vi "SRV_Select a String Dialog.vi"(10 "String List":string[](array[string]), 11 "Prompt (Select one item.)":string="Select one item.") -> (0 "Cancelled?":bool, 2 "Selected String":string)   [LabVIEW 2014]
doc: "This dialog allows the user to select exactly one string from an array of input strings.\n\nAuthor: Mike Schultz"
panel:
  in  "Cancel":bool
  in  "OK":bool
  in  "Listbox":i32(listbox)
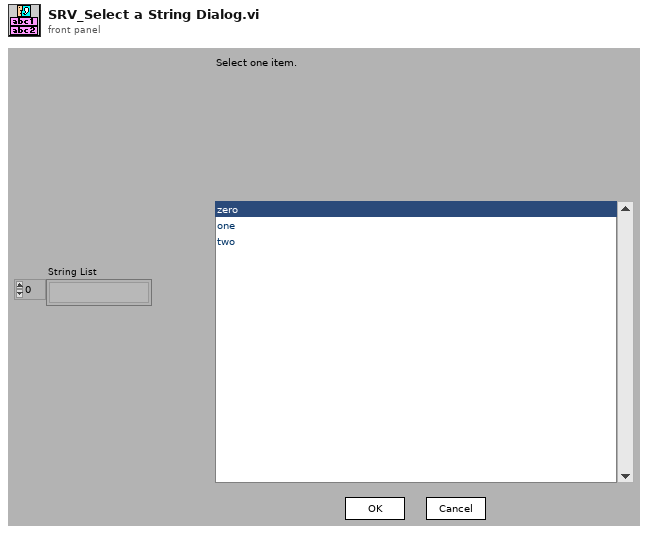
[diagram p1: front panel]
types:
  T1 = cluster{"top":i16, "left":i16, "bottom":i16, "right":i16}
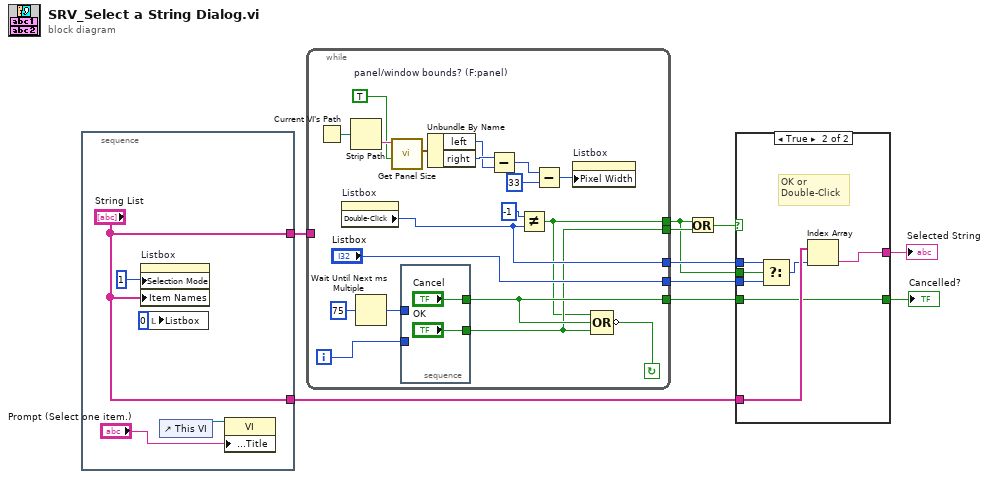
[diagram p0: block diagram]
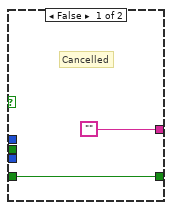
[diagram p2: hidden frame]
diagram:
  n1 = stacked-sequence {
    tunnel: ["String List"] -> w10
    tunnel: ["String List"] -> w1
    frame #0 {
      n2 = property on="Listbox" class="LstBox (strict)"("Selection Mode"=1, "Item Names"="String List") -> ()  [unwired: 2 in, 2 out]
      n3 = local write "Listbox"(0 ("Listbox")) -> ()
      n4 = control-ref of="This VI"() -> (w12:refnum<vi>)
      n5 = property class="VI"(reference=w12, "Front Panel.Title"="Prompt (Select one item.)") -> ()  [unwired: 1 in, 2 out]
    }
  }
  n6 = while {
    tunnel: w1 -> [_]
    tunnel: [w27] -> w3
    tunnel: [w26] -> w2
    tunnel: ["Listbox"] -> w6
    tunnel: [w29] -> w7
    tunnel: [w31] -> w5
    i -> [w28]
    stop <- w32 continue-if-true
    w17 = TRUE  # panel/window bounds? (F:panel)
    n7 = Current VI's Path() -> (path=w24:path)
    n8 = property on="Listbox" class="LstBox (strict)"() -> ("Double-Click"=w29:i32)  [unwired: 2 in, 2 out]
    n9 = Strip Path(path=w24) -> (name=w23:string)  [unwired: 1 out]
    n10 = Wait Until Next ms Multiple(millisecond multiple=u32 75) -> (millisecond timer value=w25:u32)
    n11 = call <vilib>:"Get Panel Size.vi"("panel/window bounds? (F:panel)"=w17, "VI name"=w23) -> ("panel location and size"=w22:T1)  [unwired: 1 in, 8 out]
    n12 = stacked-sequence {
      tunnel: ["Cancel"] -> w31
      tunnel: ["OK"] -> w27
      tunnel: w28 -> [_]
      tunnel: w25 -> [_]
      frame #0 {
      }
    }
    n13 = Unbundle By Name(w22) -> ("left"=w20:i16, "right"=w21:i16)
    n14 = Subtract(x=w21, y=w20) -> (x-y=w19:i16)
    n15 = Not Equal?(x=-1, y=w29) -> (x != y?=w26:bool)
    n16 = Subtract(x=w19, y=i16 33) -> (x-y=w16:i16)
    n17 = property on="Listbox" class="LstBox (strict)"("Pixel Width"=w16) -> ()  [unwired: 2 in, 2 out]
    n18 = Compound Arithmetic op=OR(w26, w31, w27) -> (invert w32:bool)
  }
  n19 = Or(x=w2, y=w3) -> (x .or. y?=w4:bool)
  n20 = case shown="True" w4 {
    tunnel: w10 -> [_ w45]
    tunnel: ["" w39] -> w9
    tunnel: [w37 w40] -> w8
    tunnel: w7 -> [_ w43]
    tunnel: w2 -> [_ w42]
    tunnel: w6 -> [_ w41]
    tunnel: w5 -> [w37 w40]
    frame False {
      # "Cancelled"
    }
    frame True {
      # "OK or\nDouble-Click"
      n21 = Select(t=w43, s=w42, f=w41) -> (s? t:f=w44:i32)
      n22 = Index Array(array=w45, index=w44) -> (element=w39:string)
    }
  }
  "Selected String" <- w9
  "Cancelled?" <- w8
